vi "AverageArray.vi"(10 "Samples to average":i32, 11 "Data in":dbl[](array[numeric])) -> (3 "Data out":dbl[](array[numeric]))   [LabVIEW 2019]
uses:
  <vilib>/Analysis/baseanly.llb/Mean (DBL).vi
  <vilib>/Analysis/NI_AALBase.lvlib
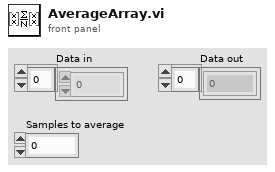
[diagram p1: front panel]
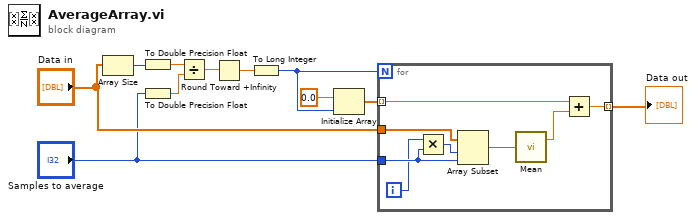
[diagram p0: block diagram]
diagram:
  n1 = Array Size(array="Data in") -> (size(s)=w1:i32)
  n2 = To Double Precision Float(number=w1) -> (double precision float=w3:dbl)
  n3 = To Double Precision Float(number="Samples to average") -> (double precision float=w4:dbl)
  n4 = Divide(x=w3, y=w4) -> (x/y=w6:dbl)
  n5 = Round Toward +Infinity(x=w6) -> (ceil(x): smallest int >= x=w5:dbl)
  n6 = To Long Integer(number=w5) -> (32bit integer=w8:i32)
  n7 = Initialize Array(0.0 ("element"), w8) -> (w9:dbl[])
  n8 = for {
    N: w8 -> [_]
    tunnel: "Samples to average" -> [w18]
    tunnel: "Data in" -> [w17]
    tunnel: w9 -> [w14] mode=indexing
    tunnel: [w12] -> w10 mode=indexing
    i -> [w15]
    n9 = Multiply(x=w15, y=w18) -> (x*y=w19:i32)
    n10 = Array Subset(array=w17, index=w19, length=w18) -> (w16:dbl[])
    n11 = call-poly <vilib>:"Mean.vi"("X"=w16) -> ("mean"=w13:dbl)  [unwired: 1 out]
    n12 = Add(x=w14, y=w13) -> (x+y=w12:dbl)
  }
  "Data out" <- w10
